vi "OLA Subtract Baseline.vi"(7 "subtract fraction":dbl=0.125, 10 "baseline":dbl[](array[numeric]), 11 "raw":dbl[](array[numeric])) -> (3 "subtracted":dbl[](array[numeric]))   [LabVIEW 2010]
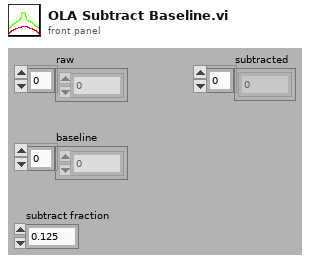
[diagram p1: front panel]
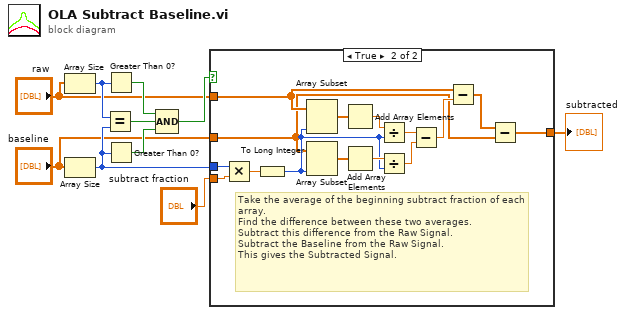
[diagram p0: block diagram]
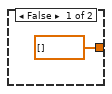
[diagram p2: hidden frame]
diagram:
  n1 = Array Size(array="raw") -> (size(s)=w10:i32)
  n2 = Array Size(array="baseline") -> (size(s)=w4:i32)
  n3 = Equal?(x=w10, y=w4) -> (x = y?=w8:bool)
  n4 = Greater Than 0?(x=w10) -> (x > 0?=w7:bool)
  n5 = Greater Than 0?(x=w4) -> (x > 0?=w9:bool)
  n6 = Compound Arithmetic op=AND(w7, w8, w9) -> (w6:bool)
  n7 = case shown="True" w6 {
    tunnel: "raw" -> [_ w16]
    tunnel: w4 -> [_ w15]
    tunnel: "subtract fraction" -> [_ w14]
    tunnel: "baseline" -> [_ w13]
    tunnel: [dbl[] [] w12] -> w1
    frame False {
    }
    frame True {
      # "Take the average of the beginning subtract fraction of each array.\nFind the difference between these two averages.\nSubtract this difference from the Raw Signal.\nSubtract the Baseline from the Raw Signal.\nThis gives the Subtracted Signal."
      n8 = Multiply(x=w15, y=w14) -> (x*y=w26:dbl)
      n9 = To Long Integer(number=w26) -> (32bit integer=w17:i32)
      n10 = Array Subset(array=w16, length=w17) -> (w25:dbl[])  [unwired: 1 in]
      n11 = Array Subset(array=w13, length=w17) -> (w24:dbl[])  [unwired: 1 in]
      n12 = Add Array Elements(numeric array=w25) -> (sum=w21:dbl)
      n13 = Add Array Elements(numeric array=w24) -> (sum=w22:dbl)
      n14 = Divide(x=w21, y=w17) -> (x/y=w20:dbl)
      n15 = Divide(x=w22, y=w17) -> (x/y=w19:dbl)
      n16 = Subtract(x=w20, y=w19) -> (x-y=w18:dbl)
      n17 = Subtract(x=w16, y=w18) -> (x-y=w23:dbl[])
      n18 = Subtract(x=w23, y=w13) -> (x-y=w12:dbl[])
    }
  }
  "subtracted" <- w1
